vi "Timestamp.vi"() -> (3 "Timestamp":string)   [LabVIEW 2021]
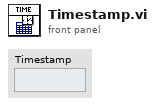
[diagram p1: front panel]
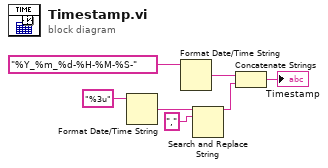
[diagram p0: block diagram]
diagram:
  n1 = Format Date/Time String(time format string (%c)="%3u") -> (date/time string=w6:string)  [unwired: 2 in]
  n2 = Format Date/Time String(time format string (%c)="%Y_%m_%d-%H-%M-%S-") -> (date/time string=w5:string)  [unwired: 2 in]
  n3 = Search and Replace String(input string=w6, search string=",") -> (result string=w7:string)  [unwired: 6 in, 3 out]
  n4 = Concatenate Strings(w5, w7) -> (→"Timestamp":string)
